vi "Compare Noise.vi"() -> ()   [LabVIEW 2021]
uses:
  <vilib>/Analysis/2dsp.llb/Decimate (single shot, DBL).vi
  <vilib>/Analysis/baseanly.llb/Mean (DBL).vi
  <vilib>/Waveform/WDTOps.llb/WDT Waveform Duration DBL.vi
  <vilib>/Waveform/WDTOps.llb/WDT Get Waveform Subset DBL.vi
  <vilib>/Utility/TDMS File Viewer/NI_TDMS File Viewer.lvlib
  <vilib>/Analysis/NI_AALPro.lvlib
  <vilib>/Analysis/NI_AALBase.lvlib
panel:
  in  "Offset":dbl[](array[numeric])=[0.0, 0.0, 0.25]
  out "Distribution":T1(graph)
  in  "intervals":i32=50
  out "actual duration":dbl=0.06998002763376732 format="%0.2f"
  out "actual start samples/time":dbl=0.010000003948809276 format="%0.2f"
  in  "Name":string[](array[string])=["NI-6376 .5V sine 1 V range", "Red Pitaya .5V sine 1 V range", "NI-5105 .25V sine .5 V range"]
  in  "Factor":dbl[](array[numeric])=[1.0, 1.14041, 1.06173]
  out "Waveform Graph":waveform(dbl)[](graph)
  in  "Desimation":i32[](array[numeric])=[1, 1, 1]
  in  "Chan":string[](array[string])=["V X1", "V X1", "V X1"]
  in  "Preview file":i32=-1
  in  "Files":path[](array[path])=[path "U:/My Documents/NHMFL/Rack set-up/Compare digitizers/6376_lockin_p004_083122.tdms", path "U:/My Documents/NHMFL/Rack set-up/Compare digitizers/RP_lockin_p002_083122.tdms", path "U:/My Documents/NHMFL/Rack set-up/Compare digitizers/5105_lockin_250mV_p011_083122.tdms"]
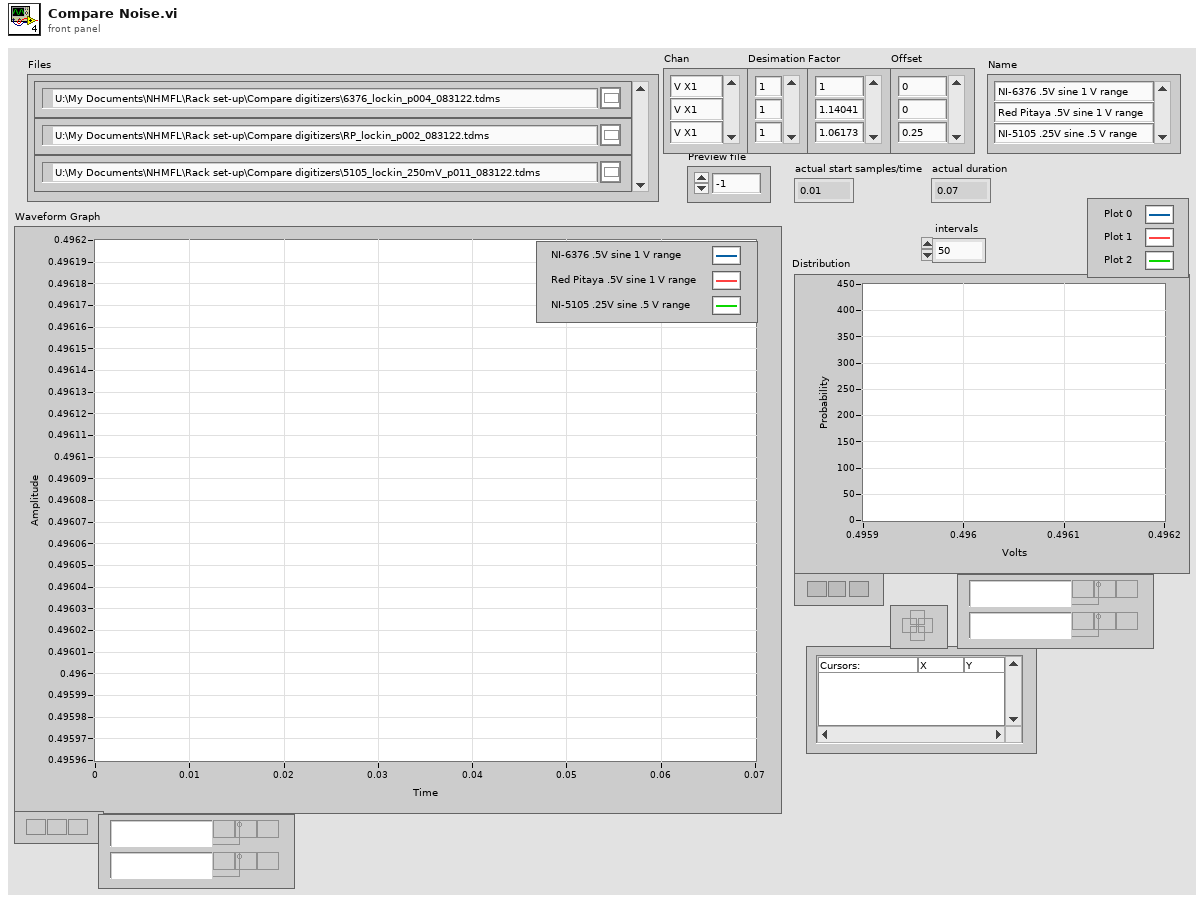
[diagram p1: front panel]
types:
  T1 = cluster{"X Values":dbl[], "Histogram: h(x)":i32[]}[]
  T2 = enum16{"open", "open or create", "create or replace", "create", "open (read-only)"}
  T3 = cluster{"X Values":dbl[], "Histogram: h(x)":i32[]}
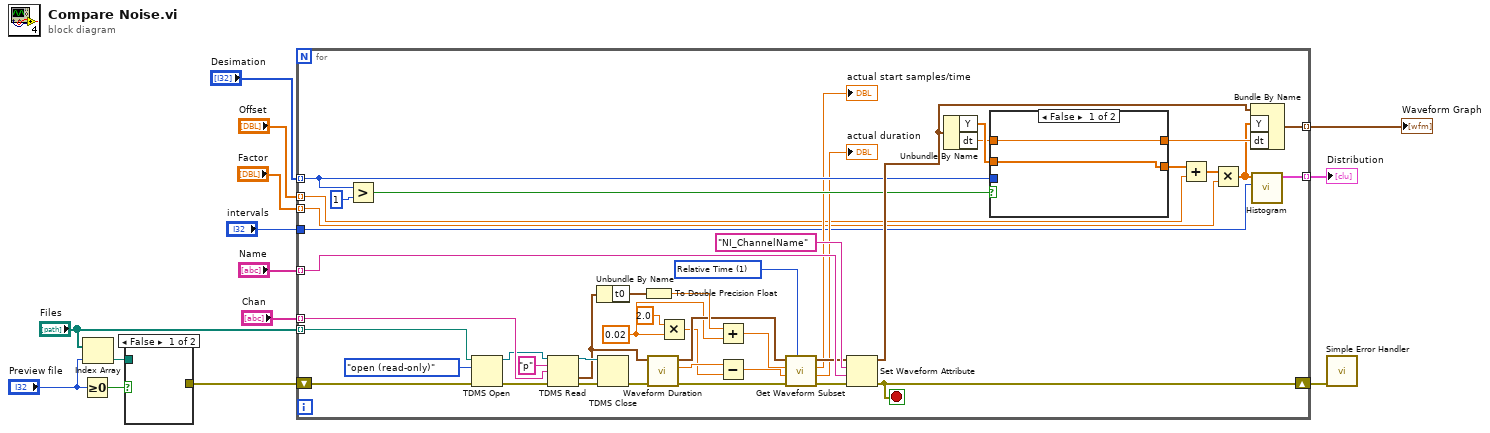
[diagram p0: block diagram]
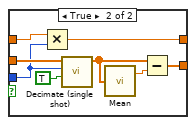
[diagram p2: hidden frame]
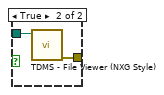
[diagram p3: hidden frame]
diagram:
  n1 = Greater Or Equal To 0?(x="Preview file") -> (x >= 0?=w13:bool)
  n2 = Index Array(array="Files", index="Preview file") -> (element=w12:path)
  n3 = case shown="False" w13 {
    tunnel: w12 -> [_ w16]
    tunnel: [_ w15] -> w9
    frame False {
    }
    frame True {
      n4 = call <vilib>:"TDMS - File Viewer (NXG Style).vi"("file in"=w16) -> ("error out"=w15:errorcluster)  [unwired: 9 in, 1 out]
    }
  }
  n5 = for {
    tunnel: "Files" -> [w60] mode=indexing
    tunnel: "Chan" -> [w55] mode=indexing
    shift-right: [w26] -> w4
    shift-left: w9 -> [w58]
    tunnel: "Desimation" -> [w43] mode=indexing
    tunnel: [w48] -> w7 mode=indexing
    tunnel: "Factor" -> [w19] mode=indexing
    tunnel: "Name" -> [w45] mode=indexing
    tunnel: "intervals" -> [w21]
    tunnel: [w20] -> w2 mode=indexing
    tunnel: "Offset" -> [w17] mode=indexing
    stop <- w26 stop-if-true
    w23 = u16 1 items=["Samples", "Relative Time"] ("start/duration format")
    w30 = 0.02 ("y")
    n6 = Greater?(x=w43, y=1) -> (0:w41:bool)
    n7 = TDMS Open(8:w58, 10:T2."open (read-only)" ("operation (0:open)"), 11:w60) -> (0:w57:errorcluster, 3:w54:refnum<k34>)  [unwired: 4 in]
    n8 = TDMS Read(0:w54, 5:"p" ("group name in"), 7:w55, 11:w57) -> (4:w52:refnum<k34>, 10:w36:waveform(dbl), 15:w53:errorcluster)  [unwired: 4 in, 3 out]
    n9 = Unbundle By Name(w36) -> ("t0"=w31:timestamp)
    n10 = TDMS Close(8:w53, 11:w52) -> (0:w34:errorcluster)  [unwired: 1 out]
    n11 = To Double Precision Float(number=w31) -> (double precision float=w38:dbl)
    n12 = call-poly <vilib>:"Waveform Duration.vi"("error in (no error)"=w34, "waveform in"=w36) -> ("error out"=w33:errorcluster, "duration"=w32:dbl, "waveform out"=w35:waveform(dbl))  [unwired: 7 in]
    n13 = Multiply(x=2.0, y=w30) -> (x*y=w29:dbl)
    n14 = Add(x=w38, y=w30) -> (x+y=w37:dbl)
    n15 = Subtract(x=w32, y=w29) -> (x-y=w27:dbl)
    n16 = call-poly <vilib>:"Get Waveform Subset.vi"("start/duration format"=w23, "error in (no error)"=w33, "duration"=w27, "start samples/time"=w37, "waveform in"=w35) -> ("error out"=w39:errorcluster, "actual duration"=→"actual duration":dbl, "actual start samples/time"=→"actual start samples/time":dbl, "waveform out"=w40:waveform(dbl))  [unwired: 1 in]
    n17 = Set Waveform Attribute(4:w39, 5:w45, 6:"NI_ChannelName" ("name"), 7:w40) -> (0:w26:errorcluster, 3:w46:waveform(dbl))  [unwired: 1 out]
    n18 = Unbundle By Name(w46) -> ("Y"=w51:dbl[], "dt"=w50:dbl)
    n19 = case shown="False" w41 {
      tunnel: w51 -> [w61 w70]
      tunnel: w50 -> [w62 w68]
      tunnel: [w62 w67] -> w49
      tunnel: [w61 w64] -> w47
      tunnel: w43 -> [_ w63]
      frame False {
      }
      frame True {
        n20 = Multiply(x=w68, y=w63) -> (x*y=w67:dbl)
        n21 = call-poly <vilib>:"Decimate (single shot).vi"("averaging"=TRUE, "decimating factor"=w63, "X"=w70) -> ("Decimated Array"=w66:dbl[])  [unwired: 7 in, 1 out]
        n22 = call-poly <vilib>:"Mean.vi"("X"=w66) -> ("mean"=w65:dbl)  [unwired: 1 out]
        n23 = Subtract(x=w66, y=w65) -> (x-y=w64:dbl[])
      }
    }
    n24 = Add(x=w47, y=w17) -> (x+y=w18:dbl[])
    n25 = Multiply(x=w18, y=w19) -> (x*y=w22:dbl[])
    n26 = Bundle By Name(cluster=w46, "Y"=w22, "dt"=w49) -> (w48:waveform(dbl))
    n27 = call <vilib>:"Histogram.vi"("intervals"=w21, "X"=w22) -> ("Histogram Graph"=w20:T3)  [unwired: 6 in, 3 out]
  }
  "Waveform Graph" <- w7
  "Distribution" <- w2
  n28 = call <vilib>:"Simple Error Handler.vi"("error in (no error)"=w4) -> ()  [unwired: 4 in, 5 out]
